vi "Force_powervi.vi"(0 "IMUS":sgl[](array[numeric])=[0.0, 0.0, 0.0, 0.0, 0.0, 0.0, 0.0, 0.0, 0.0, 0.0, 0.0, 0.0, 0.0, 0.0, 0.0, 0.0, 0.0, 0.0, 0.0, 0.0, 0.0, 0.0, 0.0, 0.0, 0.0, 0.0, 0.0, 0.0, 0.0], 5 "L_force":sgl, 7 "R_force":sgl) -> (4 "FPGA_data_out":sgl[](array[numeric]), 6 "L_force_psd":sgl, 8 "R_force_psd":sgl)   [LabVIEW 2019]
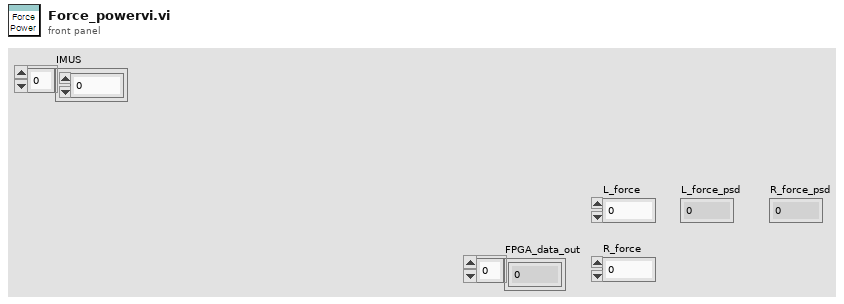
[diagram p1: front panel]
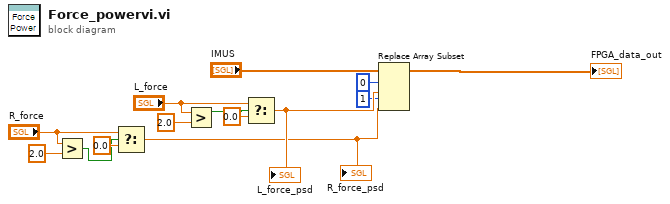
[diagram p0: block diagram]
diagram:
  n1 = Greater?(x="R_force", y=2.0) -> (0:w5:bool)
  n2 = Select(t="R_force", s=w5, f=sgl 0.0) -> (s? t:f=w8:sgl)
  "R_force_psd" <- w8
  n3 = Greater?(x="L_force", y=sgl 2.0) -> (0:w2:bool)
  n4 = Select(t="L_force", s=w2, f=sgl 0.0) -> (s? t:f=w10:sgl)
  "L_force_psd" <- w10
  n5 = Replace Array Subset(array="IMUS", new element #1=w10, index #1=0 ("인덱스"), new element #2=w8, index #2=1 ("인덱스")) -> (→"FPGA_data_out":sgl[])
